vi "Manage Collision.vi"(11 "Missile-Missile in":refnum<class "Missile-Missile.lvclass">) -> (1 "Remove GB Components out":refnum<class "Game Board Component.lvclass">[](array[class]), 2 "GB Components out":refnum<class "Game Board Component.lvclass">[](array[class]))   [LabVIEW 2021, in "Missile-Missile.lvclass"]
doc: "MIT Licence\nCopyright (c) 2024 David Grollier"
uses:
  Missile-Missile.lvclass
  C:/Users/David/Documents/GameSoccerSpace/Source/Collision/Collision.lvclass
  Game Componants/Game Board Component/Game Board Component.lvclass
  Game Componants/Game Board Component/Movable/Movable.lvclass
  C:/Users/David/Documents/GameSoccerSpace/Source/Game Componants/Game Board Component/Game Board Component.lvclass
  Collision.lvclass
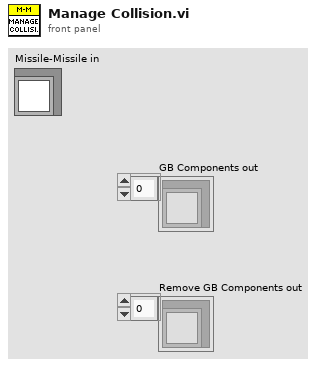
[diagram p1: front panel]
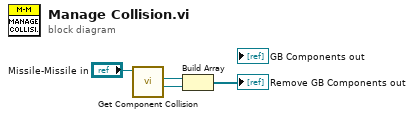
[diagram p0: block diagram]
diagram:
  n1 = call "Get Component Collision.vi"("Collision in"="Missile-Missile in") -> ("Movable out"=w2:refnum<class "Movable.lvclass">, "GB Component out"=w3:refnum<class "Game Board Component.lvclass">)  [unwired: 9 in]
  n2 = Build Array(w3, w2) -> (→"Remove GB Components out":refnum<class "Game Board Component.lvclass">[])
